vi "Delete_Folder (SubVI).vi"(8 "error in":errorcluster, 10 "String":string, 11 "AppInfo in":T1) -> (0 "error out":errorcluster, 3 "AppInfo out":T1)   [LabVIEW 2010]
uses:
  Ctl/AppInfo.ctl
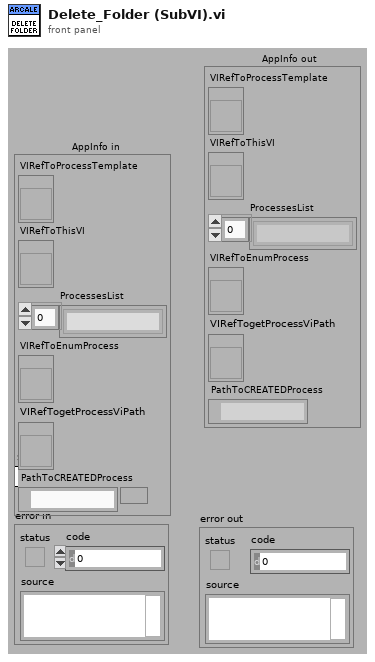
[diagram p1: front panel]
types:
  T1 = typedef "AppInfo.ctl" = cluster{"VIRefToProcessTemplate":refnum<vi>, "VIRefToThisVI":refnum<vi>, "ProcessesList":string[], "VIRefToEnumProcess":refnum<vi>, "VIRefTogetProcessViPath":refnum<vi>, "PathToCREATEDProcess":path}
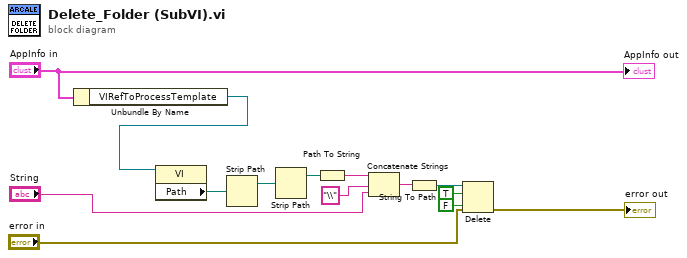
[diagram p0: block diagram]
diagram:
  n1 = Unbundle By Name("AppInfo in") -> ("VIRefToProcessTemplate"=w1:refnum<vi>)
  n2 = property class="VI"(reference=w1) -> ("Path"=w2:path)  [unwired: 1 in, 2 out]
  n3 = Strip Path(path=w2) -> (stripped path=w3:path)  [unwired: 1 out]
  n4 = Strip Path(path=w3) -> (stripped path=w5:path)  [unwired: 1 out]
  n5 = Path To String(path=w5) -> (string=w6:string)
  n6 = Concatenate Strings(w6, "\\" ("string"), "String") -> (w7:string)
  n7 = String To Path(string=w7) -> (path=w10:path)
  n8 = Delete(path (use dialog)=w10, entire hierarchy (F)=TRUE, confirm (F)=FALSE, error in="error in") -> (error out=→"error out":errorcluster)  [unwired: 1 in, 2 out]
  "AppInfo out" <- "AppInfo in"
